vi "Graphics-LTWH to LTRB.vi"(0 "Left":i16, 2 "Top":i16, 3 "Width":i16, 5 "Height":i16) -> (7 "TLRB":cluster{"Left":i16, "Top":i16, i16, i16})   [LabVIEW 2020]
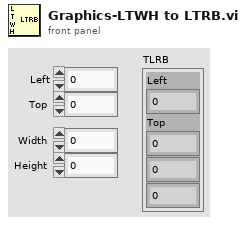
[diagram p1: front panel]
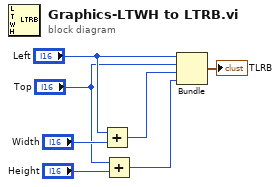
[diagram p0: block diagram]
diagram:
  n1 = Add(x="Left", y="Width") -> (x+y=w3:i16)
  n2 = Add(x="Top", y="Height") -> (x+y=w2:i16)
  n3 = Bundle("Left"="Left", "Top"="Top", w3, w2) -> (→"TLRB":cluster{"Left":i16, "Top":i16, i16, i16})  [unwired: 1 in]
